vi "timer.vi"(8 "error in (no error)":errorcluster, 11 "Action":T1) -> (0 "error out":errorcluster, 3 "Numeric":u32)   [LabVIEW 2023]
doc: "Show time elapsed"
uses:
  #typedef_action.ctl
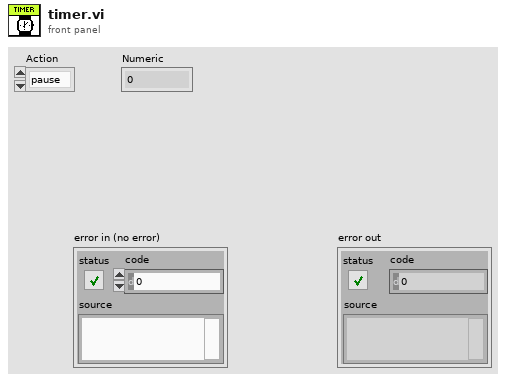
[diagram p1: front panel]
types:
  T1 = typedef "#typedef_action.ctl" = enum16{"pause", "reset", "run"}
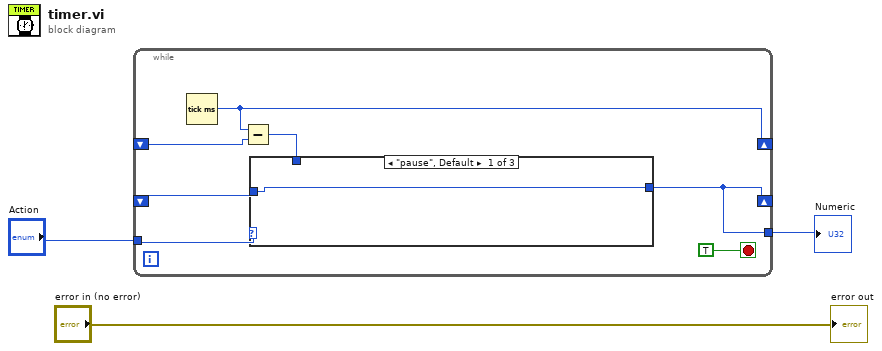
[diagram p0: block diagram]
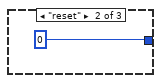
[diagram p2: hidden frame]
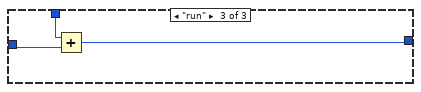
[diagram p3: hidden frame]
diagram:
  n1 = while {
    shift-right: [w7] -> _
    shift-left: _ -> [w8]
    tunnel: "Action" -> [w9]
    shift-right: [w6] -> _
    shift-left: _ -> [w5]
    tunnel: [w7] -> w3
    stop <- TRUE stop-if-true
    n2 = Tick Count (ms)() -> (millisecond timer value=w6:u32)
    n3 = Subtract(x=w6, y=w5) -> (x-y=w4:u32)
    n4 = case shown="\"pause\", Default" w9 {
      tunnel: [w11 0 w13] -> w7
      tunnel: w8 -> [w11 _ w15]
      tunnel: w4 -> [_ _ w14]
      frame "pause", Default {
      }
      frame "reset" {
      }
      frame "run" {
        n5 = Add(x=w14, y=w15) -> (x+y=w13:u32)
      }
    }
  }
  "Numeric" <- w3
  "error out" <- "error in (no error)"
